vi "Agilent DMM Wait for Operation Complete (OPC).vi"(8 "error in (no error)":errorcluster, 10 "Timeout, ms (10000)":u32=10000, 11 "VISA Resource Name":refnum<visa-resource-name>) -> (0 "error out":errorcluster, 3 "dup VISA Resource Name":refnum<visa-resource-name>)   [LabVIEW 2011]
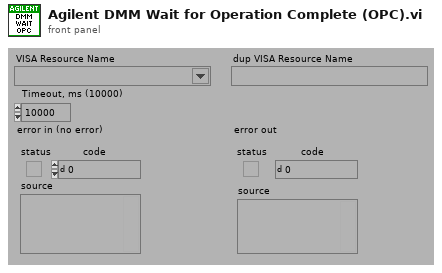
[diagram p1: front panel]
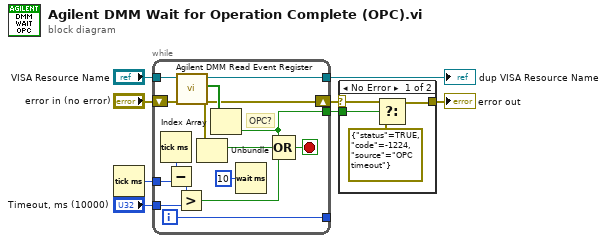
[diagram p0: block diagram]
diagram:
  n1 = Tick Count (ms)() -> (millisecond timer value=w8:u32)
  n2 = while {
    tunnel: [w14] -> w5
    tunnel: "VISA Resource Name" -> [w18]
    tunnel: "Timeout, ms (10000)" -> [w20]
    tunnel: w8 -> [w23]
    shift-right: [w15] -> w4
    shift-left: "error in (no error)" -> [w16]
    tunnel: [w10] -> w1
    tunnel: [w9] -> _
    i -> [w9]
    stop <- w11 stop-if-true
    # "OPC?"
    n3 = Tick Count (ms)() -> (millisecond timer value=w22:u32)
    n4 = Subtract(x=w22, y=w23) -> (x-y=w21:u32)
    n5 = Greater?(x=w21, y=w20) -> (0:w12:bool)
    n6 = call "Agilent DMM Read Event Register.vi"("error in (no error)"=w16, "VISA Resource Name"=w18) -> ("error out"=w15:errorcluster, "Event Register"=w17:bool[], "dup VISA Resource Name"=w10:refnum<visa-resource-name>)  [unwired: 7 out]
    n7 = Unbundle(w15) -> ("status"=w13:bool)  [unwired: 2 out]
    n8 = Index Array(array=w17) -> (element=w14:bool)  [unwired: 1 in]
    n9 = Wait (ms)(milliseconds to wait=u32 10) -> ()  [unwired: 1 out]
    n10 = Compound Arithmetic op=OR(w14, w13, w12) -> (w11:bool)
  }
  "dup VISA Resource Name" <- w1
  n11 = case shown="No Error" w4 {
    selector: w4 -> [w26 w28]
    tunnel: w5 -> [w27 _]
    tunnel: [w25 w28] -> w3
    frame No Error {
      n12 = Select(t=w26, s=w27, f=errorcluster {"status"=TRUE, "code"=-1224, "source"="OPC timeout"}) -> (s? t:f=w25:errorcluster)
    }
    frame Error {
    }
  }
  "error out" <- w3
